vi "Emergency Stop.vi"(8 "error in (no error)":errorcluster, 11 "reference in":refnum<class "Instrument.lvclass">) -> (0 "error out":errorcluster, 3 "reference out":refnum<class "Instrument.lvclass">)   [LabVIEW 2023, in "HAL GOOP4.lvlib" / "Instrument.lvclass"]
uses:
  Instrument.lvclass
  Interfaces/IConfigure/IConfigure.lvclass
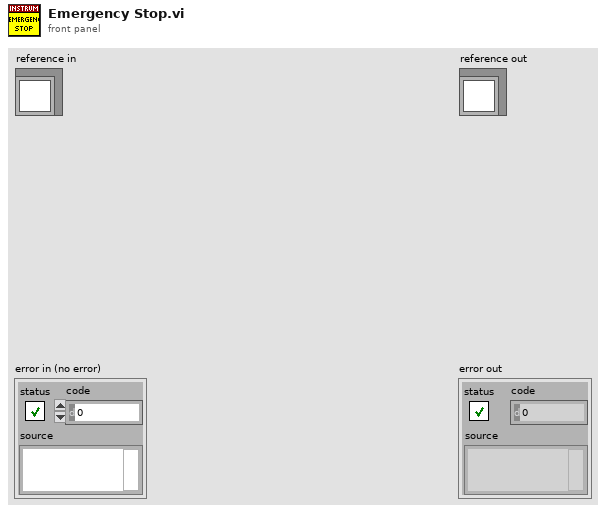
[diagram p1: front panel]
types:
  T1 = typedef "HAL GOOP4.lvlib/Instrument.lvclass/ObjectAttributes.ctl" = cluster{"IConfigure":refnum<class "IConfigure.lvclass">, "Ref Count":u8, "Start Count":u8}
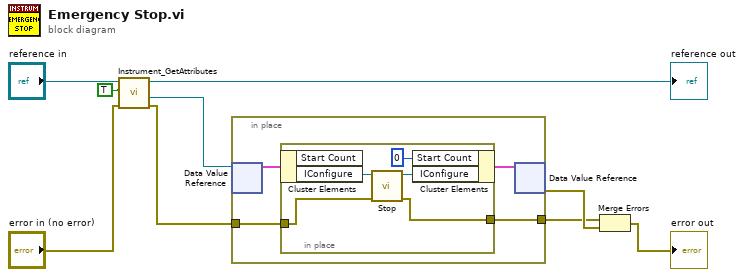
[diagram p0: block diagram]
diagram:
  n1 = call "Instrument_GetAttributes.vi"("Error In"="error in (no error)", "OnlyGetDvrReference(False)"=TRUE, "reference in"="reference in") -> ("Error Out"=w4:errorcluster, "DataRef"=w5:refnum<data-value>, "reference out"=→"reference out":refnum<class "Instrument.lvclass">)  [unwired: 5 in, 1 out]
  n2 = in-place {
    in-place-border: w4 -> [w11]
    in-place-border: [w10] -> w3
    n3 = in-place-dvr #1(w5) -> (w13:T1)  [unwired: 1 out]
    n4 = in-place {
      in-place-border: w11 -> [w16]
      in-place-border: [w15] -> w10
      n5 = in-place-cluster #2(w13) -> ("IConfigure"=w18:refnum<class "IConfigure.lvclass">)  [unwired: 1 out]
      n6 = call-dynamic "Stop.vi"("error in (no error)"=w16, "IConfigure in"=w18) -> ("error out"=w15:errorcluster, "IConfigure out"=w17:refnum<class "IConfigure.lvclass">)  [unwired: 8 in]
      n7 = in-place-cluster #2("Start Count"=u8 0, "IConfigure"=w17) -> (w12:T1)
    }
    n8 = in-place-dvr #1(w12) -> (w8:errorcluster)  [unwired: 1 out]
  }
  n9 = Merge Errors(w3, w8) -> (→"error out":errorcluster)
